vi "dat_light_sensors.vi"(7 "Timeout":i32) -> (4 "light_FR":bool, 6 "light_FL":bool, 8 "light_BR":bool, 10 "laser_L":bool, 13 "FIFO_timeout":bool, 15 "laser_R":bool)   [LabVIEW 2018]
uses:
  <vilib>/rvi/DataTransferAndStorage/Container/Common/niFpgaContainerExecOnDevCompGetState.vi
  <vilib>/rvi/Emulation/niFpgaEmulationIsFPGAContextNoSignature.vi
  <vilib>/rvi/Emulation/niFpgaSctlEmulationGetInTimedLoop.vi
  <vilib>/rvi/errors/niFpgaSetErrorForExecOnDevCompSimple.vi
  <vilib>/rvi/eio/common/nirviEmuReportErrorAndStop.vi
  <vilib>/rvi/DataTransferAndStorage/Container/Common/niFpgaContainerGetUniqueNameForEmu.vi
  <vilib>/rvi/FIFO/Fifo_Resource/nirvififoEmulationSetSize.vi
  <vilib>/rvi/FIFO/Fifo_Resource/nirviFifoEmulationQueueMgr.vi
  <instcachedir>/0/nirviFifoEmulationQueueMgr_E5CAEC123FF24DC58D834DCA3CDAA9B5.lvgen/nirviFifoEmulationQueueMgr_E5CAEC123FF24DC58D834DCA3CDAA9B5_001.vi
  <vilib>/rvi/FIFO/Fifo_Resource/nirvififoEmulationDetermineInputValidOut.vi
  <vilib>/rvi/FIFO/Fifo_Resource/nirvififoEmulationCreateLock.vi
  <vilib>/rvi/Emulation/niFpgaProcessEmulError.vi
  <vilib>/rvi/FIFO/Fifo_Resource/nirvififoEmulationObtainLock.vi
  <vilib>/rvi/FIFO/Fifo_Resource/nirvififoEmulationReleaseLock.vi
  <vilib>/rvi/occurrence/nirviWaitOnOccurrenceBase.vi
  <vilib>/rvi/errors/nirviReportUnexpectedCaseInternalError.vi
  <vilib>/rvi/errors/nirviReportUnexpectedCaseInternalError (U32).vi
  <vilib>/Utility/error.llb/Clear Errors.vi
  <vilib>/rvi/interface/RandomDataEmulation/niFpgaRandomDataHandleErrors.vi
  <vilib>/rvi/DataTransferAndStorage/Container/XNode/niFpgaContainer.xnode
  <vilib>/rvi/FIFO/Fifo_Resource/niFpgaFifoEmulationRefIn.vi
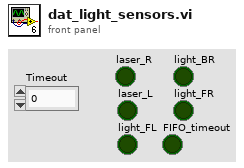
[diagram p1: front panel]
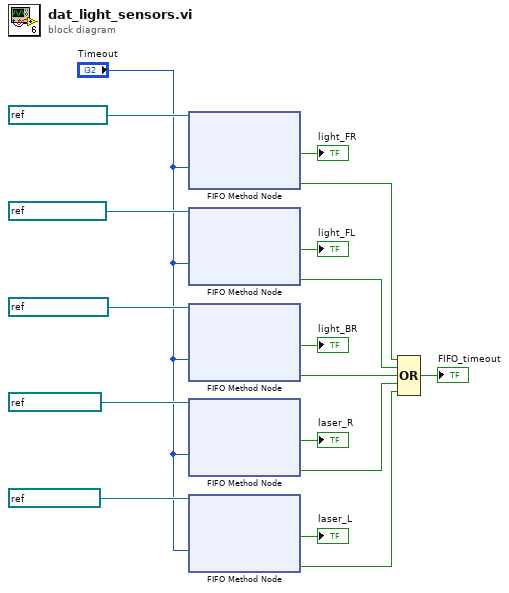
[diagram p0: block diagram]
diagram:
  n1 = xnode ("FIFO Method Node")("Timeout"="Timeout", "FIFO In"=refnum<k21> "FIFO_light_FR") -> ("Element"=→"light_FR":bool, "Timed Out?"=w11:bool)  [unwired: 1 out]
  n2 = xnode ("FIFO Method Node")("Timeout"="Timeout", "FIFO In"=refnum<k21> "FIFO_light_FL") -> ("Element"=→"light_FL":bool, "Timed Out?"=w3:bool)  [unwired: 1 out]
  n3 = xnode ("FIFO Method Node")("Timeout"="Timeout", "FIFO In"=refnum<k21> "FIFO_light_BR") -> ("Element"=→"light_BR":bool, "Timed Out?"=w8:bool)  [unwired: 1 out]
  n4 = xnode ("FIFO Method Node")("Timeout"="Timeout", "FIFO In"=refnum<k21> "FIFO_laser_R") -> ("Element"=→"laser_R":bool, "Timed Out?"=w9:bool)  [unwired: 1 out]
  n5 = xnode ("FIFO Method Node")("Timeout"="Timeout", "FIFO In"=refnum<k21> "FIFO_laser_L") -> ("Element"=→"laser_L":bool, "Timed Out?"=w10:bool)  [unwired: 1 out]
  n6 = Compound Arithmetic op=OR(w11, w3, w8, w9, w10) -> (→"FIFO_timeout":bool)
